vi "PID Integral.vi"(7 "Set? (F:Read)":bool, 8 "Error In":errorcluster, 9 "Integral (0)":dbl[unit], 11 "VISA resource name":refnum<visa-resource-name>) -> (0 "Error Out":errorcluster, 1 "Integral out":dbl[unit], 3 "dup VISA resource name":refnum<visa-resource-name>)   [LabVIEW 2011, in "MGC647C.lvlib"]
doc: "Read/Set PID integral action."
uses:
  <instrlib>/MGC647C/MGC647C.lvlib
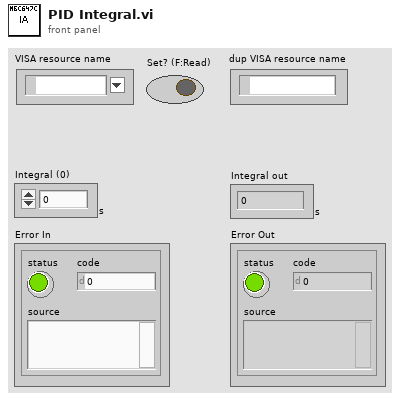
[diagram p1: front panel]
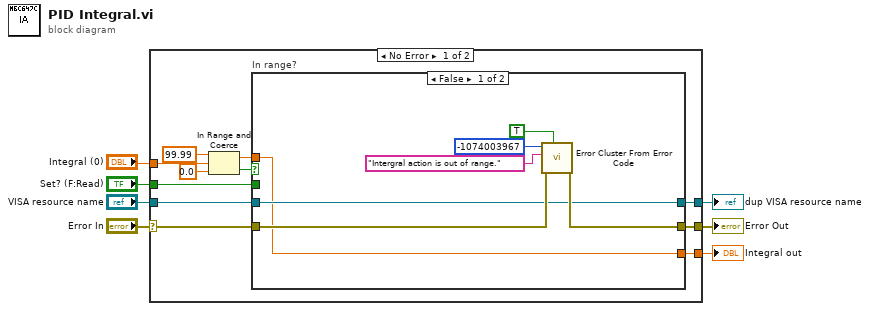
[diagram p0: block diagram]
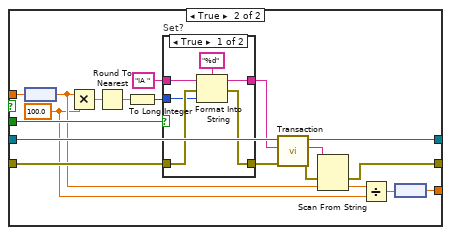
[diagram p2: hidden frame]
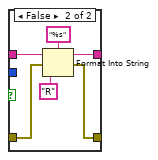
[diagram p3: hidden frame]
diagram:
  n1 = case shown="No Error" "Error In" {
    selector: "Error In" -> [w10 w58]
    tunnel: "VISA resource name" -> [w18 w57]
    tunnel: [w17 w57] -> w6
    tunnel: [w16 w58] -> w5
    tunnel: "Set? (F:Read)" -> [w15 _]
    tunnel: "Integral (0)" -> [w14 w59]
    tunnel: [w9 w59] -> w1
    frame No Error {
      n2 = In Range and Coerce(upper limit=dbl[unit] 99.99, x=w14, lower limit=dbl[unit] 0.0) -> (coerced(x)=w13:dbl[unit], In Range?=w8:bool)
      n3 = case "In range?" shown="False" w8 {
        tunnel: w18 -> [w23 w44]
        tunnel: [w23 w43] -> w17
        tunnel: [w24 w38] -> w16
        tunnel: w15 -> [_ w35]
        tunnel: w13 -> [w22 w34]
        tunnel: w10 -> [w25 w42]
        tunnel: [w22 w26] -> w9
        frame False {
          n4 = call <vilib>:"Error Cluster From Error Code.vi"("show call chain? (False)"=TRUE, "error in (no error)"=w25, "error message (\"\")"="Intergral action is out of range." ("error message (\"\")"), "error code (0)"=-1074003967) -> ("error out"=w24:errorcluster)  [unwired: 5 in]
        }
        frame True {
          w28 = 100.0 ("x")
          n5 = node(w34) -> (w33:dbl)
          n6 = Multiply(x=w33, y=w28) -> (x*y=w32:dbl)
          n7 = Round To Nearest(number=w32) -> (nearest integer value=w31:dbl)
          n8 = To Long Integer(number=w31) -> (32bit integer=w30:i32)
          n9 = case "Set?" shown="True" w35 {
            tunnel: w42 -> [w50 w56]
            tunnel: [w49 w55] -> w41
            tunnel: w30 -> [w48 _]
            tunnel: "IA " ("string (\"\")") -> [w47 w54]
            tunnel: [w46 w53] -> w36
            frame True {
              n10 = Format Into String(format string="%d", initial string=w47, error in=w50, w48) -> (resulting string=w46:string, error out=w49:errorcluster)
            }
            frame False {
              n11 = Format Into String(format string="%s", initial string=w54, error in=w56, "R") -> (resulting string=w53:string, error out=w55:errorcluster)
            }
          }
          n12 = call <instrlib>:"Transaction.vi"("Error In"=w41, "Command"=w36, "VISA resource name"=w44) -> ("Error Out"=w39:errorcluster, "Response"=w40:string, "dup VISA resource name"=w43:refnum<visa-resource-name>)  [unwired: 6 in]
          n13 = Scan From String(input string=w40, error in=w39, default 1=w33) -> (error out=w38:errorcluster, output 1=w29:dbl)  [unwired: 2 in, 2 out]
          n14 = Divide(x=w29, y=w28) -> (x/y=w27:dbl)
          n15 = node(w27) -> (w26:dbl[unit])
        }
      }
    }
    frame Error {
    }
  }
  "dup VISA resource name" <- w6
  "Error Out" <- w5
  "Integral out" <- w1
